vi "IQ.vi"(10 "Config":T1={"Ref channel index"=1, "Active channel index"=2}, 11 "array":waveform(dbl)[](array[waveform])) -> (2 "Output waveform":waveform(dbl)[](array[waveform]), 3 "Lockin output":T2 {"X" format="%#_3g"; "Y" format="%#_3g"; "R" format="%#_3g"})   [LabVIEW 2019]
doc: "This example demonstrates how to acquire a continuous amount of data (Waveform) using the DAQ device's internal clock. It also shows how to synchronize two devices for different device families (E Series, S Series, M Series, X Series, DSA, and SC Express), to simultaneously acquire the data.\n\nFor instructions on how to connect your signals to the DAQ device, refer to your device documentation."
uses:
  <vilib>/Waveform/WDTOps.llb/WDT Get Final Time Value DBL.vi
  <vilib>/Analysis/NI_AALPro.lvlib
panel:
  out "Ref waveform":waveform(dbl)[](array[waveform])
  # "Lockin"
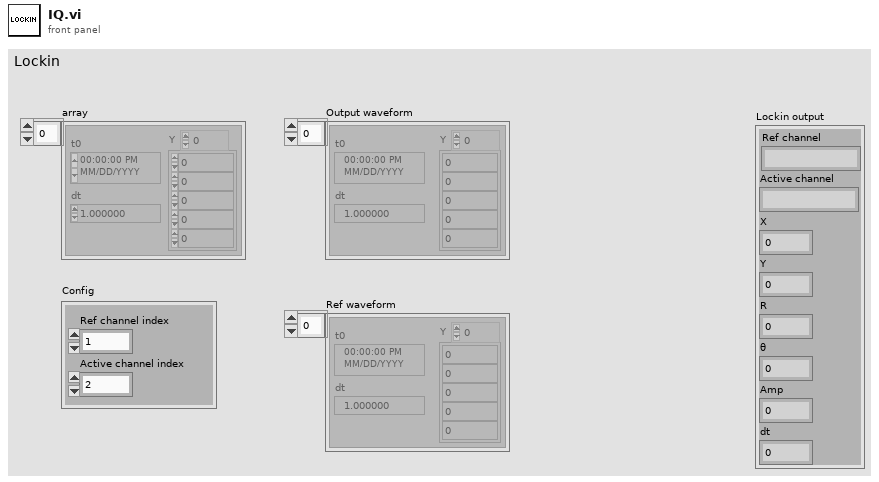
[diagram p1: front panel]
types:
  T1 = cluster{"Ref channel index":i32, "Active channel index":i32}
  T2 = cluster{"X":dbl, "Y":dbl, "R":dbl, "θ":dbl, "Amp":dbl, "dt":dbl, "Active channel":string, "Ref channel":string}
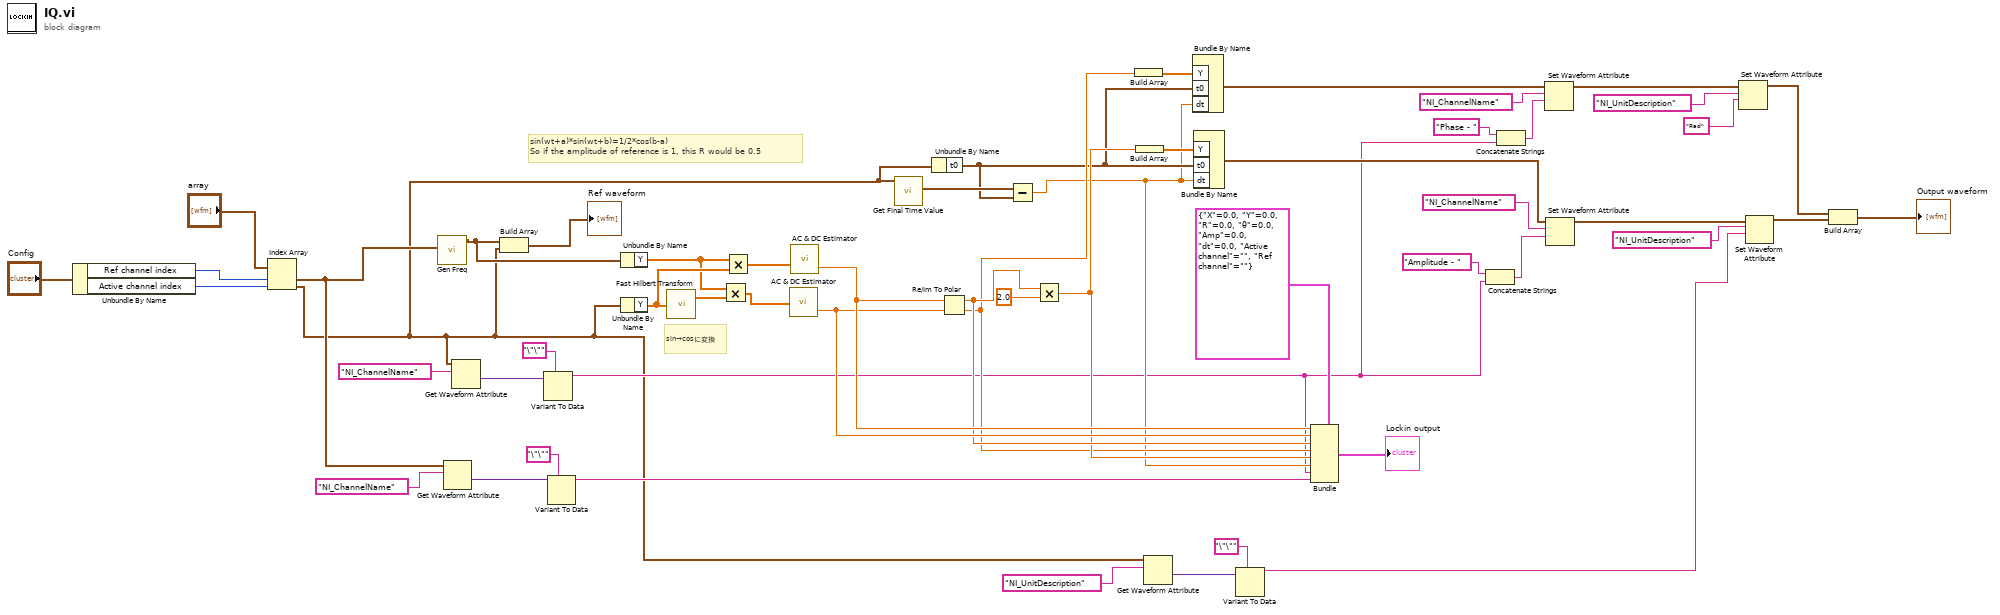
[diagram p0: block diagram]
diagram:
  # "sin(wt+a)*sin(wt+b)=1/2*cos(b-a)\nSo if the amplitude of reference is 1, this R would be 0.5"
  # "sin→cosに変換"
  n1 = Unbundle By Name("Config") -> ("Ref channel index"=w10:i32, "Active channel index"=w9:i32)
  n2 = Index Array(array="array", index #1=w10, index #2=w9) -> (element #1=w14:waveform(dbl), element #2=w1:waveform(dbl))
  n3 = call "Gen Freq.vi"("Ref"=w14) -> ("Ref_PLL_Out"=w48:waveform(dbl))  [unwired: 10 in]
  n4 = Get Waveform Attribute(6:"NI_ChannelName" ("name"), 7:w14) -> (1:w12:variant)  [unwired: 2 in, 3 out]
  n5 = Get Waveform Attribute(6:"NI_ChannelName" ("name"), 7:w1) -> (1:w18:variant)  [unwired: 2 in, 3 out]
  n6 = Build Array(w48, w1) -> (→"Ref waveform":waveform(dbl)[])
  n7 = Variant To Data(type="\"\"" ("name"), Variant=w18) -> (data=w7:string)  [unwired: 1 in, 1 out]
  n8 = Variant To Data(type="\"\"" ("name"), Variant=w12) -> (data=w6:string)  [unwired: 1 in, 1 out]
  n9 = Unbundle By Name(w48) -> ("Y"=w52:dbl[])
  n10 = Unbundle By Name(w1) -> ("Y"=w53:dbl[])
  n11 = call <vilib>:"Fast Hilbert Transform.vi"("X"=w53) -> ("Hilbert{X}"=w54:dbl[])  [unwired: 1 out]
  n12 = Multiply(x=w52, y=w54) -> (x*y=w50:dbl[])
  n13 = Multiply(x=w52, y=w53) -> (x*y=w51:dbl[])
  n14 = call <vilib>:"AC & DC Estimator.vi"("Signal (V)"=w50) -> ("DC estimate (V)"=w46:dbl)  [unwired: 1 out]
  n15 = call <vilib>:"AC & DC Estimator.vi"("Signal (V)"=w51) -> ("DC estimate (V)"=w47:dbl)  [unwired: 1 out]
  n16 = call-poly <vilib>:"Get Final Time Value.vi"("waveform in"=w1) -> ("tf"=w41:timestamp)  [unwired: 8 in, 2 out]
  n17 = Unbundle By Name(w1) -> ("t0"=w37:timestamp)
  n18 = Re/Im To Polar(2:w46, 3:w47) -> (0:w38:dbl, 1:w45:dbl)
  n19 = Subtract(x=w41, y=w37) -> (x-y=w16:dbl)
  n20 = Multiply(x=w45, y=2.0) -> (x*y=w43:dbl)
  n21 = Build Array(w38) -> (w39:dbl[])
  n22 = Build Array(w43) -> (w44:dbl[])
  n23 = Get Waveform Attribute(6:"NI_UnitDescription" ("name"), 7:w1) -> (1:w5:variant)  [unwired: 2 in, 3 out]
  n24 = Bundle By Name("Y"=w39, "t0"=w37, "dt"=w16) -> (w34:waveform(dbl))  [unwired: 1 in]
  n25 = Bundle By Name("Y"=w44, "t0"=w37, "dt"=w16) -> (w33:waveform(dbl))  [unwired: 1 in]
  n26 = Variant To Data(type="\"\"" ("name"), Variant=w5) -> (data=w2:string)  [unwired: 1 in, 1 out]
  n27 = Bundle(cluster=T2 {"X"=0.0, "Y"=0.0, "R"=0.0, "θ"=0.0, "Amp"=0.0, "dt"=0.0, "Active channel"="", "Ref channel"=""} ("Lock-in output"), "X"=w47, "Y"=w46, "R"=w45, "θ"=w38, "Amp"=w43, "dt"=w16, "Active channel"=w7, "Ref channel"=w6) -> (→"Lockin output":T2)
  n28 = Concatenate Strings("Amplitude - " ("name"), w7) -> (w28:string)
  n29 = Concatenate Strings("Phase - " ("name"), w7) -> (w29:string)
  n30 = Set Waveform Attribute(5:w29, 6:"NI_ChannelName" ("name"), 7:w34) -> (3:w24:waveform(dbl))  [unwired: 1 in, 2 out]
  n31 = Set Waveform Attribute(5:w28, 6:"NI_ChannelName" ("name"), 7:w33) -> (3:w22:waveform(dbl))  [unwired: 1 in, 2 out]
  n32 = Set Waveform Attribute(5:"Rad" ("name"), 6:"NI_UnitDescription" ("name"), 7:w24) -> (3:w23:waveform(dbl))  [unwired: 1 in, 2 out]
  n33 = Set Waveform Attribute(5:w2, 6:"NI_UnitDescription" ("name"), 7:w22) -> (3:w21:waveform(dbl))  [unwired: 1 in, 2 out]
  n34 = Build Array(w23, w21) -> (→"Output waveform":waveform(dbl)[])
